vi "WriteSDO4b.vi"(4 "data array":u8[](array[numeric])=[0, 0, 0, 0] format="%.0x", 5 "R/W":i8, 7 "Node ID":i8=1, 8 "error in":errorcluster, 9 "Sub Index":i8 format="%.0x", 10 "Index":i16 format="%.0x", 11 "ObjHandle in":T1) -> (0 "error out":errorcluster, 2 "写入数组":u8[](array[numeric]) format="%x", 3 "ObjHandle out":T1)   [LabVIEW 2019]
doc: "This VI writes a SDO message to a particular node."
uses:
  <vilib>/nican/nican.llb/xobjhandle.ctl
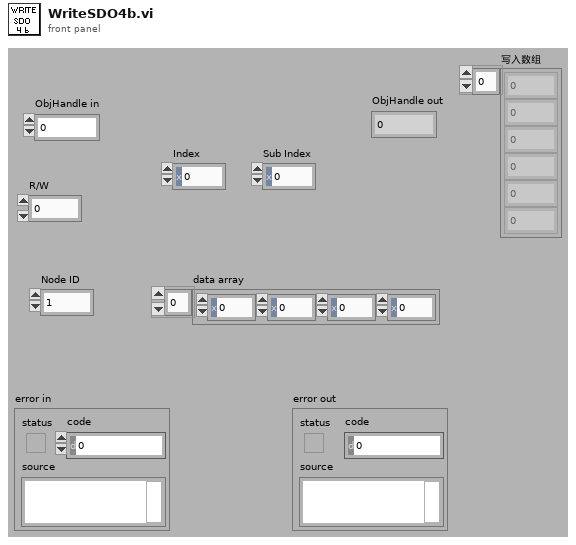
[diagram p1: front panel]
types:
  T1 = typedef "xobjhandle.ctl" = u32
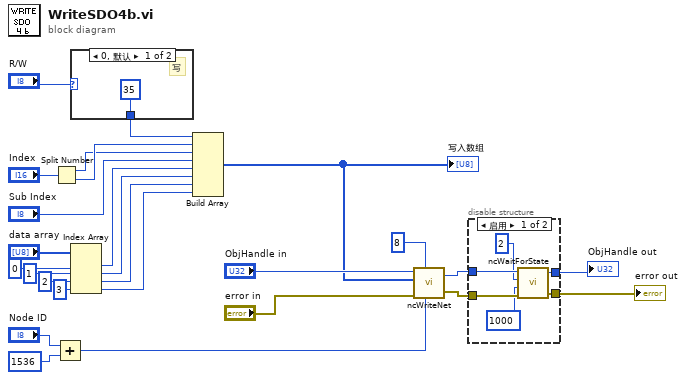
[diagram p0: block diagram]
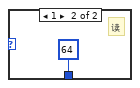
[diagram p2: hidden frame]
diagram:
  n1 = Split Number(x="Index") -> (hi(x)=w19:u8, lo(x)=w20:u8)
  n2 = Add(x="Node ID", y=u32 1536) -> (x+y=w14:u32)
  n3 = case shown="0, 默认" "R/W" {
    tunnel: [i8 35 ("元素") i8 64 ("元素")] -> w4
    frame 0, Default {
      # "写"
    }
    frame 1 {
      # "读"
    }
  }
  n4 = Index Array(array="data array", index #1=0 ("索引"), index #2=1 ("索引"), index #3=2 ("索引"), index #4=3 ("索引")) -> (element #1=w17:u8, element #2=w9:u8, element #3=w8:u8, element #4=w1:u8)
  n5 = Build Array(w4, w20, w19, "Sub Index", w17, w9, w8, w1) -> (w16:u8[])
  "写入数组" <- w16
  n6 = call <vilib>:"ncWriteNet.vi"("ArbitrationId"=w14, "DataLength"=u32 8, "Error in"="error in", "Data"=w16, "ObjHandle in"="ObjHandle in") -> ("Error out"=w13:errorcluster, "ObjHandle out"=w10:T1)  [unwired: 1 in]
  n7 = disable-structure shown="启用" {
    disable-tunnel: w13 -> [w34 w35]
    disable-tunnel: [w33 w35] -> w12
    disable-tunnel: [w32 w36] -> w11
    disable-tunnel: w10 -> [w31 w36]
    frame Enabled {
      n8 = call <vilib>:"ncWaitForState.vi"("Error in"=w34, "Timeout"=u32 1000, "DesiredState"=u32 2, "ObjHandle in"=w31) -> ("Error out"=w33:errorcluster, "ObjHandle out"=w32:T1)  [unwired: 1 out]
    }
    frame Disabled {
    }
  }
  "error out" <- w12
  "ObjHandle out" <- w11
